vi "HFRR ADV v013 new software.vi"() -> ()   [LabVIEW 2025] (continued)
                n3075 = local read "Temperature before test 3"() -> (→"Temperature after test 5":dbl)
                n3076 = local read "Temperature after test 3"() -> (→"Temperature after test 4":dbl)
                n3077 = local read "Humidity before test 3"() -> (→"Humidity before test 4":dbl)
                n3078 = local write "Temperature before test 3"(w3787) -> ()
                n3079 = local read "image data"() -> (w3778:T15)
                n3080 = String To Path(string="C:\\LAB-IQ\\im\\Temp_resized.jpg") -> (path=w3779:path)
                "path 2" <- w3779
                n3081 = call <vilib>:"Write JPEG File.vi"("image data"=w3778, "path to JPEG file"=w3779) -> ()  [unwired: 8 in, 2 out]
                "Ref A Test Date :" <- "Ref A Test Date :"
                "Ref B Test Date :" <- "Ref B Test Date :"
                "Ref B Scar Value :" <- "Ref B Scar Value :"
                "Ref A Scar Value :" <- "Ref A Scar Value :"
              }
              frame #1 {
                (unwired) HTML_Report_Image_Alignment."MIDDLE" ("alignment (default)")
                w3815 = u16 0 items=["portrait", "landscape"] ("orientation (portrait)")
                (unwired) HTML_Report_Image_Alignment."ABSMIDDLE" ("alignment (default)")
                (unwired) "TESTED BY : "
                (unwired) "TESTED DATE :"
                (unwired) "SAMPLE ID : "
                (unwired) "SAMPLE DESIGN : "
                w3848 = "\r"
                # "add image"
                n3082 = Wait (ms)(milliseconds to wait=u32 20) -> ()  [unwired: 1 out]
                n3083 = local read "Sample ID  2"() -> (w3841:string)
                n3084 = local read "Wear Scar X"() -> (w3813:dbl)
                "Length ( microns ) 2" <- w3813
                n3085 = local read "Wear Scar Y"() -> (w3812:dbl)
                "Wear Scar Y ( microns ) :" <- w3812
                n3086 = local read "Test Date 2"() -> (w3842:string)
                n3087 = local read "Tested by 2"() -> (w3843:string)
                n3088 = local read "String 46"() -> (w3839:string)
                n3089 = local read "String 48"() -> (w3845:string)
                n3090 = local read "String 47"() -> (w3844:string)
                n3091 = local read "String 49"() -> (w3846:string)
                n3092 = local read "String 10"() -> (w3799:string)
                n3093 = local read "s.NO 2"() -> (w3840:string)
                n3094 = Add(x=w3813, y=w3812) -> (x+y=w3811:dbl)
                n3095 = call <vilib>:"New Report.vi"("report type"=enum16{"Standard Report", "HTML"}."HTML") -> ("report out"=w3819:refnum<class "NI_report.lvclass">, "error out"=w3817:errorcluster)  [unwired: 13 in]
                n3096 = Concatenate Strings(w3848, w3839, w3840, w3848, w3845, w3841, w3848, w3844, w3842, w3848, w3846, w3843, w3848) -> (→"test by 2":string)
                n3097 = Concatenate Strings("C:\\LAB-IQ\\Data\\" ("string"), w3799, ".jpg" ("string")) -> ()  [unwired: 1 out]
                n3098 = Divide(x=w3811, y=2.0) -> (x/y=→"Mean Wear ( microns) :":dbl)
                n3099 = call-dynamic "Set Report Orientation.vi"("report in"=w3819, "orientation (portrait)"=w3815, "error in (no error)"=w3817) -> ("report out"=w3818:refnum<class "NI_report.lvclass">, "error out"=w3816:errorcluster)  [unwired: 11 in]
                n3100 = for {
                  N: 5 -> [_]
                  tunnel: w3818 -> [w3869]
                  tunnel: [w3868] -> w3797
                  tunnel: w3816 -> [w3867]
                  tunnel: [w3866] -> w3796
                  n3101 = call-dynamic "Set Report Tab Width.vi"("report in"=w3869, "error in (no error)"=w3867) -> ("report out"=w3868:refnum<class "NI_report.lvclass">, "error out"=w3866:errorcluster)  [unwired: 12 in]
                }
                n3102 = local read "TITTLE"() -> (w3814:string)
                n3103 = call-dynamic "Set Report Header Text.vi"("report in"=w3797, "center header text"=w3814, "error in (no error)"=w3796) -> ("report out"=w3835:refnum<class "NI_report.lvclass">, "error out"=w3834:errorcluster)  [unwired: 11 in]
                n3104 = for {
                  N: 1 -> [_]
                  tunnel: [w3873] -> w3821
                  tunnel: [w3872] -> w3820
                  tunnel: w3835 -> [w3871]
                  tunnel: w3834 -> [w3870]
                  n3105 = call-dynamic "New Report Line.vi"("report in"=w3871, "error in (no error)"=w3870) -> ("report out"=w3873:refnum<class "NI_report.lvclass">, "error out"=w3872:errorcluster)  [unwired: 12 in]
                }
                n3106 = for {
                  N: 2 -> [_]
                  tunnel: [w3865] -> w3827
                  tunnel: [w3864] -> w3826
                  tunnel: w3821 -> [w3863]
                  tunnel: w3820 -> [w3862]
                  n3107 = call-dynamic "New Report Line.vi"("report in"=w3863, "error in (no error)"=w3862) -> ("report out"=w3865:refnum<class "NI_report.lvclass">, "error out"=w3864:errorcluster)  [unwired: 12 in]
                }
                n3108 = for {
                  N: 25 -> [_]
                  tunnel: w3827 -> [w3861]
                  tunnel: w3826 -> [w3859]
                  tunnel: [w3860] -> w3830
                  tunnel: [w3858] -> w3829
                  n3109 = call-dynamic "Set Report Tab Width.vi"("report in"=w3861, "error in (no error)"=w3859) -> ("report out"=w3860:refnum<class "NI_report.lvclass">, "error out"=w3858:errorcluster)  [unwired: 12 in]
                }
                n3110 = control-ref of="Tab Control 9"() -> (w3825:refnum<vi>)
                n3111 = call-dynamic "Append Control Image to Report.vi"("report in"=w3830, "alignment (default)"=HTML_Report_Image_Alignment."ABSMIDDLE", "ctrl reference"=w3825, "error in (no error)"=w3829) -> ("report out"=w3824:refnum<class "NI_report.lvclass">, "error out"=w3823:errorcluster)  [unwired: 8 in, 2 out]
                n3112 = for {
                  N: 3 -> [_]
                  tunnel: [w3857] -> w3808
                  tunnel: [w3856] -> w3807
                  tunnel: w3824 -> [w3855]
                  tunnel: w3823 -> [w3854]
                  n3113 = call-dynamic "New Report Line.vi"("report in"=w3855, "error in (no error)"=w3854) -> ("report out"=w3857:refnum<class "NI_report.lvclass">, "error out"=w3856:errorcluster)  [unwired: 12 in]
                }
                n3114 = for {
                  N: 100 -> [_]
                  tunnel: w3808 -> [w3853]
                  tunnel: w3807 -> [w3851]
                  tunnel: [w3852] -> w3804
                  tunnel: [w3850] -> w3802
                  n3115 = call-dynamic "Set Report Tab Width.vi"("report in"=w3853, "error in (no error)"=w3851) -> ("report out"=w3852:refnum<class "NI_report.lvclass">, "error out"=w3850:errorcluster)  [unwired: 12 in]
                }
                n3116 = String To Path(string="C:\\LAB-IQ\\im\\Temp_resized.jpg") -> (path=w3794:path)
                n3117 = call-poly <vilib>:"Append Image to Report.vi"("report in"=w3804, "path or URL of image"=w3794, "error in (no error)"=w3802) -> ("report out"=w3803:refnum<class "NI_report.lvclass">, "error out"=w3801:errorcluster)  [unwired: 9 in, 2 out]
                n3118 = call-poly <vilib>:"Open HTML Report in Browser.vi"("report in"=w3803, "error in (no error)"=w3801) -> ("report out"=w3838:refnum<class "NI_report.lvclass">, "error out"=w3837:errorcluster)  [unwired: 11 in, 1 out]
                n3119 = call-dynamic "Dispose Report.vi"("report in"=w3838, "error in (no error)"=w3837) -> ()  [unwired: 13 in, 1 out]
              }
              frame #2 {
              }
              frame #3 {
                n3120 = disable-structure shown="Disabled" {
                  frame Disabled {
                    n3121 = local read "String 10"() -> (w3878:string)
                    n3122 = Concatenate Strings("C:\\LAB-IQ-NXT\\Data\\" ("string"), w3878, ".jpg" ("string")) -> (w3876:string)
                    n3123 = String To Path(string=w3876) -> (path=w3875:path)
                    n3124 = Delete(path (use dialog)=w3875) -> ()  [unwired: 4 in, 3 out]
                  }
                  frame Enabled {
                  }
                }
                n3125 = local write "Print 2"(FALSE ("Print")) -> ()
              }
            }
          }
        }
      }
    }
    n3126 = property on="SetTemp" class="DigNum (strict)"("Disabled"=w1814) -> ()  [unwired: 2 in, 2 out]
    n3127 = Multiply(x=w1804, y=w1806) -> (x*y=w1805:dbl)
    n3128 = local read "MWSD"() -> (w1803:dbl)
    n3129 = Add(x=w1805, y=w1803) -> (x+y=→"WS1.4":dbl)
    n3130 = Wait (ms)(milliseconds to wait=u32 50) -> ()  [unwired: 1 out]
    n3131 = Wait (ms)(milliseconds to wait=u32 50) -> ()  [unwired: 1 out]
    n3132 = local read "Quit"() -> (w1802:bool)
  }
  n3133 = VISA Close(VISA resource name=w52, error in (no error)=w51) -> (error out=w49:errorcluster)
  n3134 = call <vilib>:"Clear Errors.vi"("error in (no error)"=w49) -> ()  [unwired: 5 in, 2 out]
  n3135 = VISA Close(VISA resource name=w37, error in (no error)=w36) -> ()  [unwired: 1 out]
  n3136 = while {
    tunnel: [w4039] -> w46
    shift-right: [w4032] -> _
    shift-left: 0.0 -> [w4035]
    shift-right: [w4031] -> _
    shift-left: 0.0 -> [w4034]
    shift-right: [w4030] -> _
    shift-left: 400.0 ("vc_cmd") -> [w4033]
    stop <- w4039 stop-if-true
    # "PID LOGIC"
    n3137 = local read "RUN"() -> (w4037:bool)
    n3138 = local read "Auto Start Temp"() -> (w4026:bool)
    n3139 = local read "Auto Start Test"() -> (w4036:bool)
    n3140 = local read "START TEMP"() -> (w4028:bool)
    n3141 = And(x=w4026, y=w4036) -> (x .and. y?=w4027:bool)
    n3142 = Or(x=w4037, y=w4027) -> (x .or. y?=w4038:bool)
    n3143 = And(x=w4038, y=w4028) -> (x .and. y?=w4029:bool)
    n3144 = Wait (ms)(milliseconds to wait=u32 20) -> ()  [unwired: 1 out]
    n3145 = case shown="True" w4029 {
      tunnel: [400.0 ("out_vc_cmd") w4059] -> w4030
      tunnel: [w4042 w4061] -> w4031
      tunnel: [w4042 w4060] -> w4032
      tunnel: w4035 -> [_ w4050]
      tunnel: w4034 -> [_ w4049]
      tunnel: w4033 -> [_ w4048]
      frame False {
        w4042 = 0.0 ("error_out")
      }
      frame True {
        n3146 = local read "Set Strk"() -> (w4045:dbl)
        n3147 = local read "LVDT STROKE"() -> (w4043:dbl)
        n3148 = Add(x=w4045, y="Add up Stroke") -> (x+y=w4046:dbl)
        n3149 = formula code="// Zero-Hardcode Explicit Positional-Form PID Engine\n// Inputs: target_stroke, measured_stroke, dt, prev_error, integral_accumulator_in, prev_vc_cmd\n//         kp, ki, kd, max_step_change, max_amplitude, min_amplitude, startup_cmd\n// Outputs: vc_cmd, error_out, out_error, integral_accumulator_out, out_vc_cmd\n\n// 1. Calculate Tracking Error\nfloat current_error = target_stroke - measured_stroke;\nerror_out = current_error;\n\n// 2. Compute Proportional Term\nfloat p_term = kp * current_error;\n\n// 3. Compute Derivative Term\nfloat d_term = 0.0;\nif (dt > 0.0) {\n    d_term = kd * ((current_error - prev_error) / dt);\n}\n\n// 4. Update and Accumulate Integral Term\nfloat current_integral = integral_accumulator_in + (current_error * dt);\nfloat i_term = ki * current_integral;\n\n// 5. Calculate Ideal Target Command\nfloat ideal_command = startup_cmd + p_term + i_term + d_term;\n\n// 6. Anti-Windup Protection (Back-calculation method)\nif (ideal_command > max_amplitude) {\n    float excess = ideal_command - max_amplitude;\n    if (ki > 0.0) {\n        current_integral -= excess / ki;\n    }\n    ideal_command = max_amplitude;\n} else if (ideal_command < min_amplitude) {\n    float excess = ideal_command - min_amplitude;\n    if (ki > 0.0) {\n        current_integral -= excess / ki;\n    }\n    ideal_command = min_amplitude;\n}\n\n// 7. Apply Loop Rate Limiting (Protects voice coil from large voltage steps)\nfloat raw_adjustment = ideal_command - prev_vc_cmd;\n\nif (raw_adjustment > max_step_change) {\n    raw_adjustment = max_step_change;\n} else if (raw_adjustment < -max_step_change) {\n    raw_adjustment = -max_step_change;\n}\n\nfloat next_vc_cmd = prev_vc_cmd + raw_adjustment;\n\n// Final Output Safety Safeguard Clamping\nif (next_vc_cmd > max_amplitude) {\n    next_vc_cmd = max_amplitude;\n} else if (next_vc_cmd < min_amplitude) {\n    next_vc_cmd = min_amplitude;\n}\n\n// 8. Map to Shift Registers for memory persistence\nvc_cmd = next_vc_cmd;\nout_error = current_error;                     \nintegral_accumulator_out = current_integral;  \nout_vc_cmd = next_vc_cmd;"("target_stroke"=w4046, "measured_stroke"=w4043, "dt"="dt", "integral_accumulator_in"=w4049, "prev_error"=w4050, "prev_vc_cmd"=w4048, "kp"="kp", "ki"="ki", "kd"="kd", "max_step_change"="max_step_change", "max_amplitude"="max_amplitude", "min_amplitude"="min_amplitude", "startup_cmd"="startup_cmd") -> ("vc_cmd"=w4065:dbl, "out_error"=w4060:dbl, "integral_accumulator_out"=w4061:dbl, "out_vc_cmd"=w4059:dbl)  [unwired: 1 out]
        "output Vpp" <- w4065
        n3150 = Number To Fractional String(number=w4065, precision (6)=i16 1) -> (F-format string=w4063:string)  [unwired: 2 in]
        n3151 = Concatenate Strings("DAC;" ("string"), w4063) -> (w4047:string)
        n3152 = local write "Command"(w4047) -> ()
        "prev_error" <- w4050
        "integral_accumulator_in" <- w4049
        "prev_vc_cmd" <- w4048
      }
    }
    n3153 = local read "Quit"() -> (w4039:bool)
  }
  n3154 = Or(x=w42, y=w41) -> (x .or. y?=w43:bool)
  n3155 = Or(x=w39, y=w43) -> (x .or. y?=w48:bool)
  n3156 = control-ref of="new picture"() -> ()  [unwired: 1 out]
  n3157 = Or(x=w54, y=w48) -> (x .or. y?=w45:bool)
  n3158 = Or(x=w45, y=w46) -> (x .or. y?=w40:bool)
  n3159 = while {
    tunnel: [w4066] -> w53
    i -> [w4073]
    stop <- w4066 stop-if-true
    n3160 = local read "Quit"() -> (w4066:bool)
    n3161 = Equal To 0?(x=w4073) -> (x = 0?=w4071:bool)
    n3162 = call "Elapsed Time3"("Time Target (s)"=45.0, "Auto Reset"=TRUE) -> ("Time has Elapsed"=w4070:bool)  [unwired: 10 in, 7 out]
    n3163 = Wait (ms)(milliseconds to wait=u32 50) -> ()  [unwired: 1 out]
    n3164 = Or(x=w4070, y=w4071) -> (x .or. y?=w4072:bool)
    n3165 = case shown="True" w4072 {
      frame False {
      }
      frame True {
        n3166 = call <vilib>:"System Exec.vi"("run minimized? (F)"=TRUE, "error in (no error)"="error in (no error)", "command line"="powercfg.exe -change -monitor-timeout-ac 0") -> ("error out"=w4084:errorcluster)  [unwired: 5 in, 3 out]
        n3167 = call <vilib>:"System Exec.vi"("run minimized? (F)"=TRUE, "error in (no error)"=w4084, "command line"="powercfg.exe -change -disk-timeout-ac 0") -> ("error out"=w4083:errorcluster)  [unwired: 5 in, 3 out]
        n3168 = call <vilib>:"System Exec.vi"("run minimized? (F)"=TRUE, "error in (no error)"=w4083, "command line"="powercfg.exe -change -standby-timeout-ac 0") -> ("error out"=w4082:errorcluster)  [unwired: 5 in, 3 out]
        n3169 = call <vilib>:"System Exec.vi"("run minimized? (F)"=TRUE, "error in (no error)"=w4082, "command line"="powercfg.exe -change -hibernate-timeout-ac 0") -> ("error out"=w4081:errorcluster)  [unwired: 5 in, 3 out]
        n3170 = call <vilib>:"Simple Error Handler.vi"("error in (no error)"=w4081) -> ("error out"=w4087:errorcluster)  [unwired: 4 in, 4 out]
        n3171 = call <vilib>:"Clear Errors.vi"("error in (no error)"=w4087) -> ("error out"=→"error out":errorcluster)  [unwired: 5 in, 1 out]
      }
    }
  }
  n3172 = Compound Arithmetic op=OR(w56, w40, w53) -> (w55:bool)
  n3173 = flat-sequence {
    tunnel: w55 -> [_]
    tunnel: [w4089] -> w18
    tunnel: w18 -> [_]
    frame #0 {
      n3174 = call "CLOSE CONNECTION.vi"() -> ("error out"=w4089:errorcluster)  [unwired: 11 in]
    }
    frame #1 {
      n3175 = Quit LabVIEW(quit? (T)=TRUE) -> ()
      n3176 = local write "Quit"(FALSE ("EXIT")) -> ()
    }
  }
  n3177 = property on="Heater Button" class="Bool (strict)"("Visible"=TRUE) -> ()  [unwired: 2 in, 2 out]
  n3178 = disable-structure shown="Disabled" {
    disable-tunnel: _ -> [w4095 _]
    disable-tunnel: _ -> [w4092 _]
    disable-tunnel: _ -> [w4093 _]
    frame Disabled {
      n3179 = disable-structure shown="Disabled" {
        disable-tunnel: [w4102 _] -> w4094
        frame Disabled {
          n3180 = while {
            shift-right: [w4144] -> w4100
            shift-left: errorcluster {"status"=TRUE, "code"=0, "source"="Init"} ("error out") -> [w4109]
            shift-right: [w4143] -> w4099
            shift-left: _ -> [w4110]
            shift-right: [w4142] -> _
            shift-left: "" -> [w4141]
            tunnel: [w4103] -> w4102
            shift-right: ["Set Rh"] -> _
            shift-left: 0.0 ("Set Rh") -> [w4135]
            tunnel: [w4112] -> _
            i -> [w4112]
            stop <- w4103 stop-if-true
            n3181 = flat-sequence {
              tunnel: w4109 -> [w4147]
              tunnel: [w4147] -> w4108
              frame #0 {
                n3182 = Wait (ms)(milliseconds to wait=u32 200) -> ()  [unwired: 1 out]
              }
            }
            n3183 = local read "Com Port 3"() -> (w4111:refnum<visa-resource-name>)
            n3184 = local read "Humidity Str Rec"() -> (w4113:string)
            n3185 = Not Equal?(x="Set Rh", y=w4135) -> (x != y?=w4140:bool)
            n3186 = Number To Decimal String(number="Set Rh") -> (decimal integer string=w4138:string)  [unwired: 1 in]
            n3187 = Not Equal?(x=w4111, y=w4110) -> (x != y?=w4106:bool)
            n3188 = Concatenate Strings("#setPoint00" ("string"), w4138) -> (w4139:string)
            n3189 = case shown="False" w4140 {
              tunnel: w4139 -> [_ w4159]
              frame False {
                n3190 = local read "Humidity"() -> (w4156:bool)
                n3191 = case shown="True" w4156 {
                  frame False {
                    n3192 = local write "Humidity Str Send"("stop" ("Humidity Str Send")) -> ()
                  }
                  frame True {
                    n3193 = local write "Humidity Str Send"("start" ("Humidity Str Send")) -> ()
                  }
                }
              }
              frame True {
                n3194 = local write "Humidity Str Send"(w4159) -> ()
              }
            }
            n3195 = Or(x=w4106) -> (y=w4104:bool, x .or. y?=w4105:bool)
            n3196 = String Subset(string=w4113, offset (0)=7) -> (substring=w4128:string)  [unwired: 1 in]
            n3197 = Match Pattern(string=w4113, regular expression="?") -> (offset past match=w4131:i32)  [unwired: 1 in, 3 out]
            n3198 = Match Pattern(string=w4113, regular expression="v") -> (offset past match=w4134:i32)  [unwired: 1 in, 3 out]
            n3199 = case shown="True" w4105 {
              tunnel: w4108 -> [w4145 _]
              tunnel: [w4145 errorcluster {"status"=TRUE, "code"=0, "source"="Init"} ("error out")] -> w4107
              frame False {
              }
              frame True {
              }
            }
            n3200 = Equal?(x=w4131, y=-1) -> (x = y?=w4115:bool)
            n3201 = Match Pattern(string=w4128, regular expression="g") -> (after substring=w4129:string, offset past match=w4120:i32)  [unwired: 1 in, 2 out]
            n3202 = Match Pattern(string=w4128, regular expression="y") -> (after substring=w4127:string, offset past match=w4121:i32)  [unwired: 1 in, 2 out]
            n3203 = Greater?(x=w4121, y=w4120) -> (0:w4126:bool)
            n3204 = Greater Or Equal To 0?(x=w4121) -> (x >= 0?=w4118:bool)
            n3205 = Greater Or Equal To 0?(x=w4120) -> (x >= 0?=w4119:bool)
            n3206 = Or(x=w4118, y=w4119) -> (x .or. y?=w4117:bool)
            n3207 = Greater Or Equal To 0?(x=w4134) -> (x >= 0?=w4116:bool)
            n3208 = Select(t=w4127, s=w4126, f=w4129) -> (s? t:f=w4122:string)
            n3209 = case shown="Error" w4107 {
              selector: w4107 -> [w4172 w4218]
              tunnel: [w4170 w4211] -> w4144
              tunnel: w4110 -> [w4173 w4217]
              tunnel: [w4171 w4220] -> w4143
              tunnel: w4141 -> [w4160 w4219]
              tunnel: [w4167 w4219] -> w4142
              frame No Error {
                n3210 = call "Elapsed Time7"() -> ("Time has Elapsed"=w4166:bool)  [unwired: 12 in, 7 out]
                n3211 = Not Equal?(x="Humidity Str Send", y=w4160) -> (x != y?=w4162:bool)
                n3212 = Or(x=w4162, y=w4166) -> (x .or. y?=w4165:bool)
                n3213 = Select(t="Humidity Str Send", s=w4162, f="vals" ("regular expression")) -> (s? t:f=w4161:string)
                n3214 = Or(x=w4165, y="Send") -> (x .or. y?=w4169:bool)
                n3215 = case shown="True" w4169 {
                  tunnel: [w4176 w4181] -> w4170
                  tunnel: w4173 -> [w4175 w4189]
                  tunnel: w4172 -> [w4176 w4188]
                  tunnel: [w4175 w4182] -> w4171
                  tunnel: w4161 -> [_ w4187]
                  tunnel: [w4174 w4178] -> w4167
                  tunnel: "Humidity Str Send" -> [_ w4179]
                  tunnel: w4162 -> [_ w4180]
                  tunnel: w4160 -> [w4174 w4177]
                  frame False {
                  }
                  frame True {
                    n3216 = flat-sequence {
                      tunnel: w4189 -> [w4197]
                      tunnel: w4188 -> [w4196]
                      tunnel: w4187 -> [w4193]
                      tunnel: [w4195] -> w4186
                      tunnel: [w4194] -> w4185
                      tunnel: w4186 -> [w4200]
                      tunnel: w4185 -> [w4199]
                      tunnel: [w4200] -> w4184
                      tunnel: [w4199] -> w4183
                      tunnel: w4184 -> [w4207]
                      tunnel: w4183 -> [w4206]
                      tunnel: [w4205] -> w4182
                      tunnel: [w4204] -> w4181
                      frame #0 {
                        n3217 = local write "Ser Led"(TRUE ("Boolean 4")) -> ()
                        n3218 = Concatenate Strings(w4193, "\r") -> (w4192:string)
                        n3219 = VISA Write(VISA resource name=w4197, write buffer=w4192, error in (no error)=w4196) -> (VISA resource name out=w4195:refnum<visa-resource-name>, error out=w4194:errorcluster)  [unwired: 1 out]
                      }
                      frame #1 {
                        n3220 = Wait (ms)(milliseconds to wait="wait") -> ()  [unwired: 1 out]
                      }
                      frame #2 {
                        w4202 = FALSE ("Send")
                        n3221 = property class="Instr"(reference=w4207, error in=w4206) -> (reference out=w4208:refnum<visa-resource-name>, error out=w4209:errorcluster, "Serial Settings:Number of Bytes at Serial Port"=w4201:u32)
                        n3222 = local write "Send"(w4202) -> ()
                        n3223 = local write "Ser Led"(w4202) -> ()
                        n3224 = VISA Read(VISA resource name=w4208, byte count=w4201, error in (no error)=w4209) -> (VISA resource name out=w4205:refnum<visa-resource-name>, read buffer=→"Humidity Str Rec":string, error out=w4204:errorcluster)  [unwired: 1 out]
                      }
                    }
                    n3225 = Select(t=w4179, s=w4180, f=w4177) -> (s? t:f=w4178:string)
                  }
                }
              }
              frame Error {
                w4225 = u16 0 items=["None"=0, "XON/XOFF"=1, "RTS/CTS"=2, "DTR/DSR"=4] ("flow control")
                w4221 = u16 0 items=["None", "Odd", "Even", "Mark", "Space"] ("parity")
                w4224 = u16 10 items=["1.0"=10, "1.5"=15, "2.0"=20] ("stop bits")
                n3226 = VISA Close(VISA resource name=w4217, error in (no error)=w4218) -> (error out=w4216:errorcluster)
                n3227 = local write "humid"("" ("humid")) -> ()
                n3228 = local write "Humidity Str Rec"("" ("Humidity Str Rec")) -> ()
                n3229 = call <vilib>:"Clear Errors.vi"("error in (no error)"=w4216) -> ("error out"=w4215:errorcluster)  [unwired: 5 in, 1 out]
                n3230 = local read "Com Port 3"() -> (w4214:refnum<visa-resource-name>)
                n3231 = call-poly "VISA Configure Serial Port"("VISA resource name"=w4214, "timeout (10sec)"=u32 1000, "termination char\n(0xA = '\\n' = LF)"=u8 10 ("termination char\n(0xA = '\\n' = LF)"), "Enable Termination\nChar (T)"=FALSE ("Enable Termination Char (T)"), "data bits (8)"=u16 8 ("data bits"), "parity (0:none)"=w4221, "error in (no error)"=w4215, "stop bits (10: 1 bit)"=w4224, "flow control (0:none)"=w4225) -> ("VISA resource name out"=w4220:refnum<visa-resource-name>, "baud rate (9600)"=w4212:u32, "error out"=w4211:errorcluster)  [unwired: 4 in]
              }
            }
            n3232 = Compound Arithmetic op=AND(w4116, w4115, w4117) -> (w4114:bool)
            n3233 = case shown="True" w4114 {
              tunnel: w4113 -> [_ _]
              tunnel: w4122 -> [_ w4152]
              frame False {
              }
              frame True {
                w4150 = " " ("regular expression")
                n3234 = Match Pattern(string=w4152, regular expression=" ") -> (after substring=w4154:string)  [unwired: 1 in, 3 out]
                n3235 = Match Pattern(string=w4154, regular expression=w4150) -> (before substring=→"humid":string, after substring=w4151:string)  [unwired: 1 in, 2 out]
                n3236 = Match Pattern(string=w4151, regular expression=w4150) -> (before substring=→"temp_@Rh sensor":string)  [unwired: 1 in, 3 out]
              }
            }
            n3237 = local read "Quit"() -> (w4103:bool)
          }
          n3238 = VISA Close(VISA resource name=w4099, error in (no error)=w4100) -> (error out=w4096:errorcluster)
          n3239 = call <vilib>:"Clear Errors.vi"("error in (no error)"=w4096) -> ()  [unwired: 5 in, 2 out]
        }
        frame Enabled {
        }
      }
    }
    frame Enabled {
    }
  }
  n3240 = while {
    tunnel: [w4232] -> _
    i -> [w4232]
    stop <- w4228 stop-if-true
    # "Langauage selection"
    n3241 = Equal?(x="Lan flag", y=22.0) -> ()  [unwired: 1 out]
    n3242 = disable-structure shown="Disabled" {
      frame Disabled {
        n3243 = stacked-sequence {
          frame #0 {
            n3244 = case shown="\"Russian\"" "Language Selection" {
              tunnel: [0 1] -> w4234
              frame "English", Default {
              }
              frame "Russian" {
              }
            }
            n3245 = for {
              N: 130 -> [_]
              tunnel: "Table" -> [w4243]
              tunnel: w4234 -> [w4242]
              i -> [w4241]
              n3246 = Index Array(array=w4243, index (row)=w4241, index (col)=w4242) -> (element=w4240:string)
              n3247 = case shown="123" w4241 {
                tunnel: w4240 -> [w4244 w4245 _ w4246 w4247 w4248 w4249 w4250 w4251 w4252 w4253 w4254 w4255 w4256 w4257 w4258 w4259 w4260 w4261 w4262 w4263 w4264 w4265 w4266 w4267 w4268 w4269 w4270 w4271 _ _ w4272 w4273 w4274 w4275 w4276 w4277 w4286 w4293 w4300 w4307 w4311 w4314 w4317 w4319 w4321 w4322 w4323 w4324 w4325 w4326 w4327 w4328 w4329 w4330 w4331 w4332 w4333 w4334 w4335 w4336 w4337 w4338 w4339 w4340 w4341 w4342 w4343 w4344 w4345 w4346 w4347 w4348 w4349 w4350 w4351 w4352 w4353 w4354 w4355 w4356 w4357 w4358 w4359 w4360 w4361 w4362 w4363 w4364 w4365 w4366 w4367 w4368 w4369 w4370 w4371 w4372 w4373 w4374 w4375 w4376 w4377 w4378 w4379 w4380 _ w4381 w4382 w4383 w4384 w4385 w4386 w4387 w4388 w4389 w4390 w4391 w4392 w4393 _ w4394 w4395 w4396 w4397 w4398 w4399 _]
                frame 0 {
                  n3248 = local write "S"(w4244) -> ()
                }
                frame 1 {
                  n3249 = local write "S 2"(w4245) -> ()
                }
                frame 2 {
                }
                frame 3 {
                  n3250 = local write "S 4"(w4246) -> ()
                }
                frame 4 {
                  n3251 = property on="FILE" class="Str"("Caption.Text"=w4247) -> ()  [unwired: 2 in, 2 out]
                }
                frame 5 {
                  n3252 = property on="Fuel Discription :" class="Str"("Caption.Text"=w4248) -> ()  [unwired: 2 in, 2 out]
                }
                frame 6 {
                  n3253 = property on="Remarks :" class="Str"("Caption.Text"=w4249) -> ()  [unwired: 2 in, 2 out]
                }
                frame 7 {
                  n3254 = property on="Save & Continue" class="Bool (strict)"("Boolean Text.Text"=w4250) -> ()  [unwired: 2 in, 2 out]
                }
                frame 8 {
                }
                frame 9 {
                  n3255 = property on="Set Hz" class="DigNum (strict)"("Caption.Text"=w4252) -> ()  [unwired: 2 in, 2 out]
                }
                frame 10 {
                  "String 3" <- w4253
                }
                frame 11 {
                  n3256 = property on="NORMAL LOAD" class="DigNum (strict)"("Caption.Text"=w4254) -> ()  [unwired: 2 in, 2 out]
                }
                frame 12 {
                  "String 5" <- w4255
                }
                frame 13 {
                  n3257 = property on="Set Temp" class="DigNum (strict)"("Caption.Text"=w4256) -> ()  [unwired: 2 in, 2 out]
                }
                frame 14 {
                  n3258 = local write "S 15"(w4257) -> ()
                }
                frame 15 {
                  n3259 = property on="Set Rh" class="DigNum (strict)"("Caption.Text"=w4258) -> ()  [unwired: 2 in, 2 out]
                }
                frame 16 {
                  "String 13" <- w4259
                  "String 26" <- w4259
                }
                frame 17 {
                  n3260 = local write "S 18"(w4260) -> ()
                }
                frame 18 {
                  "String 17" <- w4261
                }
                frame 19 {
                  n3261 = property on="test time" class="DigNum (strict)"("Caption.Text"=w4262) -> ()  [unwired: 2 in, 2 out]
                }
                frame 20 {
                  "String 18" <- w4263
                  "String 22" <- w4263
                }
                frame 21 {
                  n3262 = property on="Elapsed time" class="DigNum (strict)"("Caption.Text"=w4264) -> ()  [unwired: 2 in, 2 out]
                }
                frame 22 {
                  n3263 = property on="Samplingtime 2" class="DigNum (strict)"("Caption.Text"=w4265) -> ()  [unwired: 2 in, 2 out]
                }
                frame 23 {
                  "String 21" <- w4266
                }
                frame 24 {
                  n3264 = property on="Countdown" class="DigNum (strict)"("Caption.Text"=w4267) -> ()  [unwired: 2 in, 2 out]
                }
                frame 25 {
                  n3265 = property on="Countdown 2" class="DigNum (strict)"("Caption.Text"=w4268) -> ()  [unwired: 2 in, 2 out]
                }
                frame 26 {
                  n3266 = property on="Engage" class="Bool (strict)"("Boolean Text.Text"=w4269) -> ()  [unwired: 2 in, 2 out]
                }
                frame 27 {
                  n3267 = property on="Boolean  4" class="Bool (strict)"("Boolean Text.Text"=w4270) -> ()  [unwired: 2 in, 2 out]
                }
                frame 28 {
                  n3268 = property on="Test \nStatus" class="Bool (strict)"("Boolean Text.Text"=w4271) -> ()  [unwired: 2 in, 2 out]
                }
                frame 29 {
                }
                frame 30 {
                }
                frame 31 {
                }
                frame 32 {
                  n3269 = property on="RSTCOF" class="Bool"("Boolean Text.Text"=w4273) -> ()  [unwired: 2 in, 2 out]
                  n3270 = property on="RST FF" class="Bool"("Boolean Text.Text"=w4273) -> ()  [unwired: 2 in, 2 out]
                  n3271 = property on="RST TEMP" class="Bool"("Boolean Text.Text"=w4273) -> ()  [unwired: 2 in, 2 out]
                  n3272 = property on="RSTV1 3" class="Bool"("Boolean Text.Text"=w4273) -> ()  [unwired: 2 in, 2 out]
                  n3273 = property on="rstv2" class="Bool"("Boolean Text.Text"=w4273) -> ()  [unwired: 2 in, 2 out]
                  n3274 = property on="RSTV1 2" class="Bool"("Boolean Text.Text"=w4273) -> ()  [unwired: 2 in, 2 out]
                  n3275 = property on="RST CP" class="Bool"("Boolean Text.Text"=w4273) -> ()  [unwired: 2 in, 2 out]
                }
                frame 33 {
                  "S 61" <- w4274
                }
                frame 34 {
                  "String 23" <- w4275
                }
                frame 35 {
                  n3276 = property on="Rh Before" class="DigNum (strict)"("Caption.Text"=w4276) -> ()  [unwired: 2 in, 2 out]
                }
                frame 36 {
                  n3277 = Match Pattern(string=w4277, regular expression=",") -> (before substring=→"bs":string, after substring=→"as":string)  [unwired: 1 in, 2 out]
                  n3278 = property on="Rh After" class="DigNum (strict)"("Caption.Text"=w4277) -> ()  [unwired: 2 in, 2 out]
                }
                frame 37 {
                  n3279 = Match Pattern(string=w4286, regular expression=",") -> (before substring=w4285:string, after substring=w4284:string)  [unwired: 1 in, 2 out]
                  "bs" <- w4285
                  "as" <- w4284
                  n3280 = Concatenate Strings(w4285, w4284) -> (w4281:string)
                  n3281 = property on="Humidity before test 2" class="DigNum (strict)"("Caption.Text"=w4281) -> ()  [unwired: 2 in, 2 out]
                  n3282 = property on="Humidity before test" class="DigNum (strict)"("Caption.Text"=w4281) -> ()  [unwired: 2 in, 2 out]
                  n3283 = Concatenate Strings(w4281, "=" ("string")) -> (w4282:string)
                  n3284 = local write "S 38"(w4282) -> ()
                }
                frame 38 {
                  n3285 = Match Pattern(string=w4293, regular expression=",") -> (before substring=w4292:string, after substring=w4291:string)  [unwired: 1 in, 2 out]
                  "bs" <- w4292
                  "as" <- w4291
                  n3286 = Concatenate Strings(w4292, w4291) -> (w4288:string)
                  n3287 = property on="Humidity after test 2" class="DigNum (strict)"("Caption.Text"=w4288) -> ()  [unwired: 2 in, 2 out]
                  n3288 = Concatenate Strings(w4288, "=" ("string")) -> (w4290:string)
                  n3289 = property on="Humidity after test" class="DigNum (strict)"("Caption.Text"=w4288) -> ()  [unwired: 2 in, 2 out]
                  n3290 = local write "S 39"(w4290) -> ()
                }
                frame 39 {
                  n3291 = Match Pattern(string=w4300, regular expression=",") -> (before substring=w4299:string, after substring=w4298:string)  [unwired: 1 in, 2 out]
                  "bs" <- w4299
                  "as" <- w4298
                  n3292 = Concatenate Strings(w4299, w4298) -> (w4295:string)
                  n3293 = property on="Temperature before test 2" class="DigNum (strict)"("Caption.Text"=w4295) -> ()  [unwired: 2 in, 2 out]
                  n3294 = property on="Temperature before test" class="DigNum (strict)"("Caption.Text"=w4295) -> ()  [unwired: 2 in, 2 out]
                  n3295 = Concatenate Strings(w4295, "=" ("string")) -> (→"String 34":string)
                }
                frame 40 {
                  n3296 = Match Pattern(string=w4307, regular expression=",") -> (before substring=w4306:string, after substring=w4305:string)  [unwired: 1 in, 2 out]
                  "bs" <- w4306
                  "as" <- w4305
                  n3297 = Concatenate Strings(w4306, w4305) -> (w4302:string)
                  n3298 = property on="Temperature after test 2" class="DigNum (strict)"("Caption.Text"=w4302) -> ()  [unwired: 2 in, 2 out]
                  n3299 = Concatenate Strings(w4302, "=" ("string")) -> (→"String 35":string)
                  n3300 = property on="Temperature after test" class="DigNum (strict)"("Caption.Text"=w4302) -> ()  [unwired: 2 in, 2 out]
                }
                frame 41 {
                  n3301 = property on="AVP" class="DigNum (strict)"("Caption.Text"=w4311) -> ()  [unwired: 2 in, 2 out]
                  n3302 = property on="AVP 2" class="DigNum (strict)"("Caption.Text"=w4311) -> ()  [unwired: 2 in, 2 out]
                  n3303 = Concatenate Strings(w4311, "=" ("string")) -> (→"String 36":string)
                }
                frame 42 {
                  n3304 = property on="MWSD" class="DigNum (strict)"("Caption.Text"=w4314) -> ()  [unwired: 2 in, 2 out]
                  n3305 = property on="MWSD 2" class="DigNum (strict)"("Caption.Text"=w4314) -> ()  [unwired: 2 in, 2 out]
                  n3306 = Concatenate Strings(w4314, "=" ("string")) -> (→"String 37":string)
                }
                frame 43 {
                  n3307 = property on="HCF 2" class="DigNum (strict)"("Caption.Text"=w4317) -> ()  [unwired: 2 in, 2 out]
                  n3308 = property on="HCF" class="DigNum (strict)"("Caption.Text"=w4317) -> ()  [unwired: 2 in, 2 out]
                  n3309 = Concatenate Strings(w4317, "=" ("string")) -> (→"String 38":string)
                }
                frame 44 {
                  n3310 = Concatenate Strings(w4319, "=" ("string")) -> (→"String 39":string)
                  n3311 = property on="WS1.4 2" class="DigNum (strict)"("Caption.Text"=w4319) -> ()  [unwired: 2 in, 2 out]
                  n3312 = property on="WS1.4" class="DigNum (strict)"("Caption.Text"=w4319) -> ()  [unwired: 2 in, 2 out]
                }
                frame 45 {
                  n3313 = property on="Save Results" class="Bool (strict)"("Boolean Text.Text"=w4321) -> ()  [unwired: 2 in, 2 out]
                }
                frame 46 {
                  n3314 = local write "S 47"(w4322) -> ()
                }
                frame 47 {
                  n3315 = local write "S 48"(w4323) -> ()
                }
                frame 48 {
                  n3316 = local write "S 49"(w4324) -> ()
                }
                frame 49 {
                  n3317 = local write "S 50"(w4325) -> ()
                }
                frame 50 {
                  n3318 = local write "S 51"(w4326) -> ()
                }
                frame 51 {
                  n3319 = local write "S 52"(w4327) -> ()
                }
                frame 52 {
                  n3320 = local write "S 53"(w4328) -> ()
                }
                frame 53 {
                  n3321 = local write "S 54"(w4329) -> ()
                }
                frame 54 {
                  n3322 = local write "S 55"(w4330) -> ()
                }
                frame 55 {
                  n3323 = local write "S 56"(w4331) -> ()
                }
                frame 56 {
                  n3324 = local write "S 57"(w4332) -> ()
                }
                frame 57 {
                  n3325 = local write "S 58"(w4333) -> ()
                }
                frame 58 {
                  n3326 = local write "S 59"(w4334) -> ()
                }
                frame 59 {
                  n3327 = local write "S 60"(w4335) -> ()
                }
                frame 60 {
                  n3328 = local write "S 62"(w4336) -> ()
                }
                frame 61 {
                  n3329 = local write "S 63"(w4337) -> ()
                }
                frame 62 {
                  n3330 = local write "S 64"(w4338) -> ()
                }
                frame 63 {
                  n3331 = local write "S 65"(w4339) -> ()
                }
                frame 64 {
                  n3332 = local write "S 66"(w4340) -> ()
                }
                frame 65 {
                  n3333 = local write "S 67"(w4341) -> ()
                }
                frame 66 {
                  n3334 = local write "S 68"(w4342) -> ()
                }
                frame 67 {
                  n3335 = local write "S 69"(w4343) -> ()
                }
                frame 68 {
                  n3336 = local write "S 70"(w4344) -> ()
                }
                frame 69 {
                  n3337 = local write "S 71"(w4345) -> ()
                }
                frame 70 {
                  n3338 = local write "S 72"(w4346) -> ()
                }
                frame 71 {
                  n3339 = local write "S 73"(w4347) -> ()
                }
                frame 72 {
                  n3340 = local write "S 74"(w4348) -> ()
                }
                frame 73 {
                  n3341 = local write "S 75"(w4349) -> ()
                }
                frame 74 {
                  n3342 = local write "S 76"(w4350) -> ()
                }
                frame 75 {
                  n3343 = local write "S 77"(w4351) -> ()
                }
                frame 76 {
                  n3344 = local write "S 78"(w4352) -> ()
                }
                frame 77 {
                  n3345 = local write "S 79"(w4353) -> ()
                }
                frame 79 {
                  n3346 = property on="Sample Temperature ( °C )" class="XYGraph (strict)"("Y Scale.Name Label.Text"=w4354) -> ()  [unwired: 2 in, 2 out]
                }
                frame 80 {
                  n3347 = local write "S 81"(w4355) -> ()
                  n3348 = property on="Humidity ( %RH )" class="XYGraph (strict)"("Y Scale.Name Label.Text"=w4355) -> ()  [unwired: 2 in, 2 out]
                }
                frame 78 {
                  n3349 = property on="Air Temperature  ( °C )" class="XYGraph (strict)"("X Scale.Name Label.Text"=w4356) -> ()  [unwired: 2 in, 2 out]
                  n3350 = property on="Humidity ( %RH )" class="XYGraph (strict)"("X Scale.Name Label.Text"=w4356) -> ()  [unwired: 2 in, 2 out]
                  n3351 = property on="Sample Temperature ( °C )" class="XYGraph (strict)"("X Scale.Name Label.Text"=w4356) -> ()  [unwired: 2 in, 2 out]
                  n3352 = property on="Coefficient Of Friction" class="XYGraph (strict)"("X Scale.Name Label.Text"=w4356) -> ()  [unwired: 2 in, 2 out]
                }
                frame 81 {
                  n3353 = property on="Air Temperature  ( °C )" class="XYGraph (strict)"("Y Scale.Name Label.Text"=w4357) -> ()  [unwired: 2 in, 2 out]
                }
                frame 82 {
                  n3354 = local write "S 84"(w4358) -> ()
                }
                frame 83 {
                  n3355 = local write "S 85"(w4359) -> ()
                }
                frame 84 {
                  n3356 = local write "S 86"(w4360) -> ()
                }
                frame 85 {
                  n3357 = local write "S 87"(w4361) -> ()
                }
                frame 86 {
                  n3358 = local write "S 88"(w4362) -> ()
                }
                frame 87 {
                }
                frame 88 {
                  n3359 = local write "S 90"(w4364) -> ()
                }
                frame 89 {
                  n3360 = local write "S 91"(w4365) -> ()
                }
                frame 90 {
                  n3361 = local write "S 92"(w4366) -> ()
                }
                frame 91 {
                  n3362 = local write "S 93"(w4367) -> ()
                }
                frame 92 {
                  n3363 = local write "S 94"(w4368) -> ()
                }
                frame 93 {
                  n3364 = local write "S 95"(w4369) -> ()
                }
                frame 94 {
                  n3365 = local write "S 96"(w4370) -> ()
                }
                frame 95 {
                  n3366 = local write "S 97"(w4371) -> ()
                }
                frame 96 {
                  n3367 = local write "S 98"(w4372) -> ()
                }
                frame 97 {
                  n3368 = local write "S 99"(w4373) -> ()
                }
                frame 98 {
                  n3369 = local write "S 100"(w4374) -> ()
                }
                frame 99 {
                  n3370 = local write "S 101"(w4375) -> ()
                }
                frame 100 {
                  n3371 = local write "S 102"(w4376) -> ()
                }
                frame 101 {
                  n3372 = local write "S 103"(w4377) -> ()
                }
                frame 102 {
                  n3373 = local write "S 104"(w4378) -> ()
                }
                frame 103 {
                  n3374 = local write "S 105"(w4379) -> ()
                }
                frame 104 {
                  n3375 = local write "S 106"(w4380) -> ()
                }
                frame 105 {
                }
                frame 106 {
                  n3376 = property on="OK Button 17" class="Bool (strict)"("Boolean Text.Text"=w4381) -> ()  [unwired: 2 in, 2 out]
                }
                frame 107 {
                  n3377 = property on="OK Button 16" class="Bool (strict)"("Boolean Text.Text"=w4382) -> ()  [unwired: 2 in, 2 out]
                }
                frame 108 {
                  n3378 = property on="TITTLE" class="Str"("Caption.Text"=w4383) -> ()  [unwired: 2 in, 2 out]
                }
                frame 109 {
                  "String 30" <- w4384
                }
                frame 110 {
                  n3379 = property on="Test Date" class="Str"("Caption.Text"=w4385) -> ()  [unwired: 2 in, 2 out]
                  "String 31" <- w4385
                }
                frame 111 {
                  n3380 = property on="Sample ID" class="Str"("Caption.Text"=w4386) -> ()  [unwired: 2 in, 2 out]
                  "String 32" <- w4386
                }
                frame 112 {
                  n3381 = property on="Tested by" class="Str"("Caption.Text"=w4387) -> ()  [unwired: 2 in, 2 out]
                  "String 33" <- w4387
                }
                frame 113 {
                  n3382 = property on="System Configured Printers 2" class="Arr (strict)"("Caption.Text"=w4388) -> ()  [unwired: 2 in, 2 out]
                }
                frame 114 {
                  n3383 = property on="Selected Printer" class="Str"("Caption.Text"=w4389) -> ()  [unwired: 2 in, 2 out]
                }
                frame 115 {
                  n3384 = property on="Select Printer 3" class="DigNum (strict)"("Caption.Text"=w4390) -> ()  [unwired: 2 in, 2 out]
                }
                frame 116 {
                  n3385 = property on="Print" class="Bool (strict)"("Boolean Text.Text"=w4391) -> ()  [unwired: 2 in, 2 out]
                }
                frame 117 {
                  "String 41" <- w4392
                }
                frame 118 {
                  n3386 = property on="tested by" class="Str"("Caption.Text"=w4393) -> ()  [unwired: 2 in, 2 out]
                }
                frame 119 {
                }
                frame 120 {
                  n3387 = property on="Export" class="Bool (strict)"("Boolean Text.Text"=w4394) -> ()  [unwired: 2 in, 2 out]
                }
                frame 121 {
                  n3388 = property on="TEMP INTERCEPT:" class="DigNum (strict)"("Caption.Text"=w4395) -> ()  [unwired: 2 in, 2 out]
                }
                frame 122 {
                  n3389 = property on="AIR TEMP INTERCEPT:" class="DigNum (strict)"("Caption.Text"=w4396) -> ()  [unwired: 2 in, 2 out]
                }
                frame 123 {
                  n3390 = property on="Select File Type" class="Enum (strict)"("Caption.Text"=w4397) -> ()  [unwired: 2 in, 2 out]
                }
                frame 124 {
                  n3391 = property on="s.NO" class="Str"("Caption.Text"=w4398) -> ()  [unwired: 2 in, 2 out]
                  "String 45" <- w4398
                }
                frame 125 {
                  n3392 = property on="trip1 8" class="Bool (strict)"("Boolean Text.Text"=w4399) -> ()  [unwired: 2 in, 2 out]
                }
                frame 126, Default {
                }
              }
            }
          }
          frame #1 {
            w4407 = TRUE ("Visible")
            n3393 = local read "S 91"() -> (w4424:string)
            n3394 = local read "S 90"() -> (w4423:string)
            n3395 = local read "S 88"() -> (w4422:string)
            n3396 = property on="File Path" class="Path"("Caption.Text"=w4423) -> ()  [unwired: 2 in, 2 out]
            n3397 = property on="SrvM CP" class="Bool (strict)"("Boolean Text.Text"=w4422) -> ()  [unwired: 2 in, 2 out]
            n3398 = local read "S 71"() -> (w4417:string)
            n3399 = local read "S 86"() -> (w4419:string)
            n3400 = local read "S 85"() -> (w4420:string)
            n3401 = local read "S 87"() -> (w4418:string)
            n3402 = local read "S 84"() -> (w4421:string)
            n3403 = local read "S 103"() -> (w4406:string)
            n3404 = local read "S 104"() -> (w4405:string)
            n3405 = property on="ENTER THE NEW PASSWORD" class="Str"("Caption.Text"=w4418) -> ()  [unwired: 2 in, 2 out]
            n3406 = property on="Password" class="Str"("Caption.Text"=w4420) -> ()  [unwired: 2 in, 2 out]
            n3407 = property on="ENTER CURRENT PASSWORD" class="Str"("Caption.Text"=w4419) -> ()  [unwired: 2 in, 2 out]
            n3408 = property on="EDIT" class="Bool (strict)"("Boolean Text.Text"=w4417) -> ()  [unwired: 2 in, 2 out]
            n3409 = property on="SAVE" class="Bool (strict)"("Boolean Text.Text"=w4421) -> ()  [unwired: 2 in, 2 out]
            n3410 = Build Array(w4406, w4405) -> (w4404:string[])
            n3411 = property on="Heater Button" class="Bool (strict)"("Strings [4]"=w4404) -> ()  [unwired: 2 in, 2 out]
            n3412 = property on="CH-HUMIDITY WET" class="DigNum (strict)"("Caption.Size to Text?"=w4407) -> ()  [unwired: 2 in, 2 out]
            n3413 = property on="CH-HUMIDITY DRY" class="DigNum (strict)"("Caption.Size to Text?"=w4407) -> ()  [unwired: 2 in, 2 out]
            n3414 = property on="CH-POWER -" class="DigNum (strict)"("Caption.Size to Text?"=w4407) -> ()  [unwired: 2 in, 2 out]
            n3415 = property on="CH-HEATER" class="DigNum (strict)"("Caption.Size to Text?"=w4407) -> ()  [unwired: 2 in, 2 out]
            n3416 = property on="CH-POWER +" class="DigNum (strict)"("Caption.Size to Text?"=w4407) -> ()  [unwired: 2 in, 2 out]
            n3417 = local read "S 92"() -> (w4416:string)
            n3418 = local read "S 93"() -> (w4415:string)
            n3419 = local read "S 105"() -> (w4402:string)
            n3420 = local read "S 106"() -> (w4401:string)
            n3421 = Build Array(w4416, w4415) -> ()  [unwired: 1 out]
            n3422 = Build Array(w4402, w4401) -> (w4403:string[])
            n3423 = local read "S 95"() -> (w4413:string)
            n3424 = local read "S 94"() -> (w4414:string)
            n3425 = local read "bs"() -> (w4429:string)
            n3426 = local read "as"() -> (w4430:string)
            n3427 = property on="Humidity" class="Bool (strict)"("Strings [4]"=w4403) -> ()  [unwired: 2 in, 2 out]
            n3428 = Concatenate Strings(w4429, "\r", w4430) -> ()  [unwired: 1 out]
            n3429 = property on="STROKE GAIN :" class="DigNum (strict)"("Caption.Text"=w4413) -> ()  [unwired: 2 in, 2 out]
            n3430 = property on="DISPLACEMENT :" class="DigNum (strict)"("Caption.Text"=w4414) -> ()  [unwired: 2 in, 2 out]
            n3431 = property on="Rh After" class="DigNum (strict)"("Caption.Size to Text?"=TRUE ("Caption.Size to Text")) -> ()  [unwired: 2 in, 2 out]
            n3432 = local read "S 48"() -> (w4453:string)
            n3433 = local read "S 50"() -> (w4451:string)
            n3434 = local read "S 51"() -> (w4450:string)
            n3435 = local read "S 49"() -> (w4452:string)
            n3436 = local read "S 52"() -> (w4449:string)
            n3437 = local read "as"() -> (w4434:string)
            n3438 = local read "bs"() -> (w4435:string)
            n3439 = local read "S 56"() -> (w4448:string)
            n3440 = local read "S 57"() -> (w4447:string)
            n3441 = local read "S 58"() -> (w4446:string)
            n3442 = local read "S 59"() -> (w4445:string)
            n3443 = property on="OPEN" class="Bool (strict)"("Boolean Text.Text"=w4449) -> ()  [unwired: 2 in, 2 out]
            n3444 = property on="OPEN 1" class="Bool (strict)"("Boolean Text.Text"=w4453) -> ()  [unwired: 2 in, 2 out]
            n3445 = property on="OPEN 2" class="Bool (strict)"("Boolean Text.Text"=w4452) -> ()  [unwired: 2 in, 2 out]
            n3446 = property on="OPEN 3" class="Bool (strict)"("Boolean Text.Text"=w4451) -> ()  [unwired: 2 in, 2 out]
            n3447 = property on="OPEN 4" class="Bool (strict)"("Boolean Text.Text"=w4450) -> ()  [unwired: 2 in, 2 out]
            n3448 = Concatenate Strings(w4435, "\r", w4434) -> ()  [unwired: 1 out]
            n3449 = local read "S 102"() -> (w4408:string)
            n3450 = property on="КОФ1" class="DigNum (strict)"("Caption.Text"=w4448) -> ()  [unwired: 2 in, 2 out]
            n3451 = local read "S 98"() -> (w4412:string)
            n3452 = local read "S 99"() -> (w4411:string)
            n3453 = local read "S 100"() -> (w4410:string)
            n3454 = local read "S 101"() -> (w4409:string)
            n3455 = property on="КОФ2" class="DigNum (strict)"("Caption.Text"=w4447) -> ()  [unwired: 2 in, 2 out]
            n3456 = property on="КОФ3" class="DigNum (strict)"("Caption.Text"=w4446) -> ()  [unwired: 2 in, 2 out]
            n3457 = property on="КОФ4" class="DigNum (strict)"("Caption.Text"=w4445) -> ()  [unwired: 2 in, 2 out]
            n3458 = local read "bs"() -> (w4433:string)
            n3459 = local read "as"() -> (w4432:string)
            n3460 = property on="CH-POWER +" class="DigNum (strict)"("Caption.Text"=w4412) -> ()  [unwired: 2 in, 2 out]
            n3461 = property on="CH-POWER -" class="DigNum (strict)"("Caption.Text"=w4411) -> ()  [unwired: 2 in, 2 out]
            n3462 = property on="CH-HEATER" class="DigNum (strict)"("Caption.Text"=w4410) -> ()  [unwired: 2 in, 2 out]
            n3463 = property on="CH-HUMIDITY DRY" class="DigNum (strict)"("Caption.Text"=w4409) -> ()  [unwired: 2 in, 2 out]
            n3464 = property on="CH-HUMIDITY WET" class="DigNum (strict)"("Caption.Text"=w4408) -> ()  [unwired: 2 in, 2 out]
            n3465 = local read "S 60"() -> (w4444:string)
            n3466 = local read "S 54"() -> (w4454:string)
            n3467 = Concatenate Strings(w4433, "\r", w4432) -> ()  [unwired: 1 out]
            n3468 = Concatenate Strings(w4454, w4444) -> ()  [unwired: 1 out]
            n3469 = local read "S 77"() -> (→"String 43":string)
            n3470 = local read "S 76"() -> (w4427:string)
            n3471 = local read "S 78"() -> (w4426:string)
            n3472 = local read "S 71"() -> (w4438:string)
            n3473 = local read "S 66"() -> (w4443:string)
            n3474 = local read "S 67"() -> (w4442:string)
            n3475 = local read "S 68"() -> (w4441:string)
            n3476 = local read "S 69"() -> (w4440:string)
            n3477 = local read "S 70"() -> (w4439:string)
            n3478 = property on="AIR TEMP" class="DigNum (strict)"("Caption.Text"=w4426) -> ()  [unwired: 2 in, 2 out]
            n3479 = property on="Set Strk" class="DigNum (strict)"("Caption.Text"=w4427) -> ()  [unwired: 2 in, 2 out]
            n3480 = property on="FRIC. FORCE :" class="DigNum (strict)"("Caption.Text"=w4443) -> ()  [unwired: 2 in, 2 out]
            n3481 = property on="TEMPERATURE :" class="DigNum (strict)"("Caption.Text"=w4442) -> ()  [unwired: 2 in, 2 out]
            n3482 = property on="SPEED OUT:" class="DigNum (strict)"("Caption.Text"=w4441) -> ()  [unwired: 2 in, 2 out]
            n3483 = property on="AIR TEMPERATURE :" class="DigNum (strict)"("Caption.Text"=w4440) -> ()  [unwired: 2 in, 2 out]
            n3484 = property on="HUMIDITY:" class="DigNum (strict)"("Caption.Text"=w4439) -> ()  [unwired: 2 in, 2 out]
            n3485 = property on="EDIT" class="Bool (strict)"("Boolean Text.Text"=w4438) -> ()  [unwired: 2 in, 2 out]
            n3486 = local read "S 79"() -> (w4425:string)
          }
          frame #2 {
          }
        }
        n3487 = local write "Lan flag"(10.0 ("Lan flag")) -> ()
      }
      frame Enabled {
      }
    }
    n3488 = Wait (ms)(milliseconds to wait=u32 2000) -> ()  [unwired: 1 out]
    n3489 = local read "Quit"() -> (w4228:bool)
  }
  n3490 = disable-structure shown="Disabled" {
    frame Disabled {
      n3491 = while {
        tunnel: [w4456] -> _
        i -> [w4456]
        stop <- w4455 continue-if-true
        n3492 = Wait (ms)(milliseconds to wait=u32 50) -> ()  [unwired: 1 out]
        n3493 = stacked-sequence {
          frame #0 {
            # "Controls Text color"
            # "Controls BG color"
            n3494 = property on="FILE" class="Str"("Text.Text Colors:Text Color"="SC  Text") -> ()  [unwired: 2 in, 2 out]
            n3495 = property on="Fuel Discription :" class="Str"("Text.Text Colors:Text Color"="SC  Text") -> ()  [unwired: 2 in, 2 out]
            n3496 = property on="tested by" class="Str"("Text.Text Colors:Text Color"="SC  Text") -> ()  [unwired: 2 in, 2 out]
            n3497 = property on="Remarks :" class="Str"("Text.Text Colors:Text Color"="SC  Text") -> ()  [unwired: 2 in, 2 out]
            n3498 = property class="DigNum (strict)"("Numeric Text.Text Colors:BG Color"="NC BG") -> ()  [unwired: 2 in, 2 out]
            n3499 = property class="DigNum (strict)"("Numeric Text.Text Colors:BG Color"="NC BG") -> ()  [unwired: 2 in, 2 out]
            n3500 = property class="DigNum (strict)"("Numeric Text.Text Colors:BG Color"="NC BG") -> ()  [unwired: 2 in, 2 out]
            n3501 = property class="DigNum (strict)"("Numeric Text.Text Colors:BG Color"="NC BG") -> ()  [unwired: 2 in, 2 out]
            n3502 = property class="DigNum (strict)"("Numeric Text.Text Colors:BG Color"="NC BG") -> ()  [unwired: 2 in, 2 out]
            n3503 = property class="DigNum (strict)"("Numeric Text.Text Colors:BG Color"="NC BG") -> ()  [unwired: 2 in, 2 out]
            n3504 = property class="DigNum (strict)"("Numeric Text.Text Colors:BG Color"="NC BG") -> ()  [unwired: 2 in, 2 out]
            n3505 = property class="DigNum (strict)"("Numeric Text.Text Colors:BG Color"="NC BG") -> ()  [unwired: 2 in, 2 out]
            n3506 = property class="DigNum (strict)"("Numeric Text.Text Colors:BG Color"="NC BG") -> ()  [unwired: 2 in, 2 out]
            n3507 = property class="DigNum (strict)"("Numeric Text.Text Colors:BG Color"="NC BG") -> ()  [unwired: 2 in, 2 out]
            n3508 = property class="DigNum (strict)"("Numeric Text.Text Colors:BG Color"="NC BG") -> ()  [unwired: 2 in, 2 out]
            n3509 = property class="DigNum (strict)"("Numeric Text.Text Colors:BG Color"="NC BG") -> ()  [unwired: 2 in, 2 out]
            n3510 = property on="FILE" class="Str"("Text.Text Colors:BG Color"="SC BG 3") -> ()  [unwired: 2 in, 2 out]
            n3511 = property on="Fuel Discription :" class="Str"("Text.Text Colors:BG Color"="SC BG 3") -> ()  [unwired: 2 in, 2 out]
            n3512 = property on="tested by" class="Str"("Text.Text Colors:BG Color"="SC BG 3") -> ()  [unwired: 2 in, 2 out]
            n3513 = property on="Remarks :" class="Str"("Text.Text Colors:BG Color"="SC BG 3") -> ()  [unwired: 2 in, 2 out]
            n3514 = property class="DigNum (strict)"("Numeric Text.Text Colors:Text Color"="NC Text") -> ()  [unwired: 2 in, 2 out]
            n3515 = property class="DigNum (strict)"("Numeric Text.Text Colors:Text Color"="NC Text") -> ()  [unwired: 2 in, 2 out]
            n3516 = property class="DigNum (strict)"("Numeric Text.Text Colors:Text Color"="NC Text") -> ()  [unwired: 2 in, 2 out]
            n3517 = property class="DigNum (strict)"("Numeric Text.Text Colors:Text Color"="NC Text") -> ()  [unwired: 2 in, 2 out]
            n3518 = property class="DigNum (strict)"("Numeric Text.Text Colors:Text Color"="NC Text") -> ()  [unwired: 2 in, 2 out]
            n3519 = property class="DigNum (strict)"("Numeric Text.Text Colors:Text Color"="NC Text") -> ()  [unwired: 2 in, 2 out]
            n3520 = property class="DigNum (strict)"("Numeric Text.Text Colors:Text Color"="NC Text") -> ()  [unwired: 2 in, 2 out]
            n3521 = property class="DigNum (strict)"("Numeric Text.Text Colors:Text Color"="NC Text") -> ()  [unwired: 2 in, 2 out]
            n3522 = property class="DigNum (strict)"("Numeric Text.Text Colors:Text Color"="NC Text") -> ()  [unwired: 2 in, 2 out]
            n3523 = property class="DigNum (strict)"("Numeric Text.Text Colors:Text Color"="NC Text") -> ()  [unwired: 2 in, 2 out]
            n3524 = property class="DigNum (strict)"("Numeric Text.Text Colors:Text Color"="NC Text") -> ()  [unwired: 2 in, 2 out]
            n3525 = property class="DigNum (strict)"("Numeric Text.Text Colors:Text Color"="NC Text") -> ()  [unwired: 2 in, 2 out]
            n3526 = property class="DigNum (strict)"("Numeric Text.Text Colors:Text Color"="NI Text  2") -> ()  [unwired: 2 in, 2 out]
            n3527 = property class="DigNum (strict)"("Numeric Text.Text Colors:Text Color"="NI Text  2") -> ()  [unwired: 2 in, 2 out]
            n3528 = property class="DigNum (strict)"("Numeric Text.Text Colors:Text Color"="NI Text  2") -> ()  [unwired: 2 in, 2 out]
            n3529 = property class="DigNum (strict)"("Numeric Text.Text Colors:Text Color"="NI Text  2") -> ()  [unwired: 2 in, 2 out]
            n3530 = property class="DigNum (strict)"("Numeric Text.Text Colors:Text Color"="NI Text  2") -> ()  [unwired: 2 in, 2 out]
            n3531 = property class="DigNum (strict)"("Numeric Text.Text Colors:Text Color"="NI Text  2") -> ()  [unwired: 2 in, 2 out]
            n3532 = property class="DigNum (strict)"("Numeric Text.Text Colors:Text Color"="NI Text  2") -> ()  [unwired: 2 in, 2 out]
            n3533 = property class="DigNum (strict)"("Numeric Text.Text Colors:Text Color"="NI Text  2") -> ()  [unwired: 2 in, 2 out]
            n3534 = property class="DigNum (strict)"("Numeric Text.Text Colors:Text Color"="NI Text  2") -> ()  [unwired: 2 in, 2 out]
            n3535 = property class="DigNum (strict)"("Numeric Text.Text Colors:Text Color"="NI Text  2") -> ()  [unwired: 2 in, 2 out]
            n3536 = property class="DigNum (strict)"("Numeric Text.Text Colors:Text Color"="NI Text  2") -> ()  [unwired: 2 in, 2 out]
            n3537 = property class="DigNum (strict)"("Numeric Text.Text Colors:Text Color"="NI Text  2") -> ()  [unwired: 2 in, 2 out]
            n3538 = property class="DigNum (strict)"("Numeric Text.Text Colors:Text Color"="NI Text  2") -> ()  [unwired: 2 in, 2 out]
